vi "local.Abort Session.vi"(8 "error in (no error)":errorcluster, 11 "SLSC Local in":refnum<class "SLSC Interface.lvclass">) -> (0 "error out":errorcluster, 3 "SLSC Local out":refnum<class "SLSC Interface.lvclass">)   [LabVIEW 2016, in "SLSC Interface.lvclass"]
uses:
  SLSC Interface Class/SLSC Interface.lvclass
  SLSC Interface Class/Read session.vi
  SLSC Interface Class/Write session.vi
  <vilib>/SLSC/SLSC.lvlib
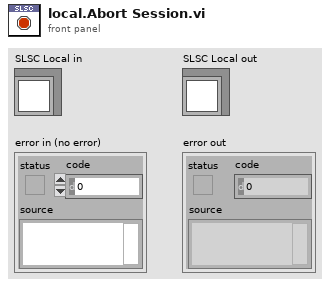
[diagram p1: front panel]
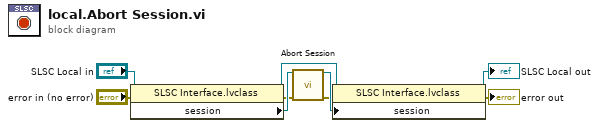
[diagram p0: block diagram]
diagram:
  n1 = property class="SLSC Interface.lvclass"(reference="SLSC Local in", error in="error in (no error)") -> (reference out=w7:refnum<class "SLSC Interface.lvclass">, error out=w3:errorcluster, "session"=w6:refnum<k21>)
  n2 = call <vilib>:"Abort Session.vi"("session in"=w6, "error in (no error)"=w3) -> ("session out"=w5:refnum<k21>, "error out"=w2:errorcluster)  [unwired: 12 in]
  n3 = property class="SLSC Interface.lvclass"(reference=w7, error in=w2, "session"=w5) -> (reference out=→"SLSC Local out":refnum<class "SLSC Interface.lvclass">, error out=→"error out":errorcluster)
